vi "Move.vi"(8 "error in (no error)":errorcluster, 9 "point(x,y)":cluster{"x":i16, "y":i16}, 10 "Tools":T8=enum."Ellipse", 11 "Data in":T1={"Class"={"Ants"=refnum, "Layer"=refnum, "Templates"=refnum, "Icon"=refnum, "Glyph"=refnum, "Settings"=refnum, "Tools"=refnum, "History"=refnum}, "Ref"={"Add Layer"=refnum, "Remove Layer"=refnum, "Line Text"=[], "Body Text Spec"=refnum, "DNL_Font"=refnum, "glyph path str"=refnum, "templates path str"=refnum, "Arrow Up"=refnum, "Arrow Down"=refnum, "IE VI Ref"=refnum, "Glyphs tree"=refnum, "Templates tree"=refnum, "Layer Icon Text"=refnum, "Layer Template"=refnum, "Body Text"=refnum, "Search Templates"=refnum, "TextMarker"=refnum, "Tab Control"=refnum, "Search Glyphs"=refnum, "Line Color"=refnum, "DNL_Glyphs []"=refnum, "Fill Color"=refnum, "Tools"=refnum, "Icon"=refnum, "Preview"=refnum, "Ants"=refnum, "Terminals"=refnum, "menu reference"=refnum, "LayerNames"=[], "GlyphLoadAnimation"=refnum, "TemplateLoadAnimation"=refnum, "refreshGlyphs"=refnum, "refreshTemplates"=refnum}, "Support"={"AntsRect"={"left"=0, "top"=0, "right"=0, "bottom"=0}, "Mouse Move Coords"={"Horizontal"=0, "Vertical"=0}, "Mouse Down Coords"={"Horizontal"=0, "Vertical"=0}, "Temp Coord"={"Horizontal"=0, "Vertical"=0}, "Action"=enum."Default", "Edge Color"=4914962, "Fill Color"=16860, "Mouse Down?"=FALSE, "Draft Mode?"=FALSE, "Temp Icon"=bytes[3102], "CTRL Pressed"=FALSE, "Move Selection?"=FALSE, "AntsRect Orig"={"left"=0, "top"=0, "right"=0, "bottom"=0}, "Text"="", "TM Set?"=FALSE, "Mouse inside icon?"=FALSE, "Tool (old value)"=0, "Pencil Move Color"=0, "Swap Colors?"=FALSE, "Shift pressed?"=FALSE}}) -> (0 "error out":errorcluster, 1 "Origin":T5, 2 "Active Layer":i32, 3 "Data out":T1={"Class"={"Ants"=refnum, "Layer"=refnum, "Templates"=refnum, "Icon"=refnum, "Glyph"=refnum, "Settings"=refnum, "Tools"=refnum, "History"=refnum}, "Ref"={"Add Layer"=refnum, "Remove Layer"=refnum, "Line Text"=[], "Body Text Spec"=refnum, "DNL_Font"=refnum, "glyph path str"=refnum, "templates path str"=refnum, "Arrow Up"=refnum, "Arrow Down"=refnum, "IE VI Ref"=refnum, "Glyphs tree"=refnum, "Templates tree"=refnum, "Layer Icon Text"=refnum, "Layer Template"=refnum, "Body Text"=refnum, "Search Templates"=refnum, "TextMarker"=refnum, "Tab Control"=refnum, "Search Glyphs"=refnum, "Line Color"=refnum, "DNL_Glyphs []"=refnum, "Fill Color"=refnum, "Tools"=refnum, "Icon"=refnum, "Preview"=refnum, "Ants"=refnum, "Terminals"=refnum, "menu reference"=refnum, "LayerNames"=[], "GlyphLoadAnimation"=refnum, "TemplateLoadAnimation"=refnum, "refreshGlyphs"=refnum, "refreshTemplates"=refnum}, "Support"={"AntsRect"={"left"=0, "top"=0, "right"=0, "bottom"=0}, "Mouse Move Coords"={"Horizontal"=0, "Vertical"=0}, "Mouse Down Coords"={"Horizontal"=0, "Vertical"=0}, "Temp Coord"={"Horizontal"=0, "Vertical"=0}, "Action"=enum."Default", "Edge Color"=4914962, "Fill Color"=16860, "Mouse Down?"=FALSE, "Draft Mode?"=FALSE, "Temp Icon"=bytes[3102], "CTRL Pressed"=FALSE, "Move Selection?"=FALSE, "AntsRect Orig"={"left"=0, "top"=0, "right"=0, "bottom"=0}, "Text"="", "TM Set?"=FALSE, "Mouse inside icon?"=FALSE, "Tool (old value)"=0, "Pencil Move Color"=0, "Swap Colors?"=FALSE, "Shift pressed?"=FALSE}})   [LabVIEW 2020, in "Tools Paint.lvclass"]
uses:
  Tools Paint.lvclass
  Ants/Ants.lvclass
  FakedArray/FakedArray.lvclass
  vi.lib/LabVIEW Icon API/lv_icon/Classes/Icon/Icon.lvclass
  Icon Library/Glyph.lvclass
  Settings/Settings.lvclass
  vi.lib/LabVIEW Icon API/lv_icon/Classes/Layer/Layer.lvclass
  Tools Paint.lvclass/Tools Paint.ctl
  Controls/Circle.ctl
  Controls/Dropper.ctl
  Controls/FCircle.ctl
  Controls/Fill.ctl
  Controls/FRect.ctl
  Controls/Line.ctl
  Controls/Move.ctl
  Controls/Pen.ctl
  Controls/IERect.ctl
  Controls/Rubber.ctl
  Controls/Selection.ctl
  Controls/Text.ctl
  Controls/Tools.ctl
  <vilib>/Utility/miscctls.llb/LVPoint32TypeDef.ctl
  Controls/SupportClass_Action.ctl
  vi.lib/LabVIEW Icon API/lv_icon/Controls/IEColor.ctl
  Controls/Support Cluster.ctl
  lv_icon.lvlib
  Controls/References Cluster.ctl
  Controls/IE Classes.ctl
  Controls/Global Data.ctl
  History/History/History.lvclass
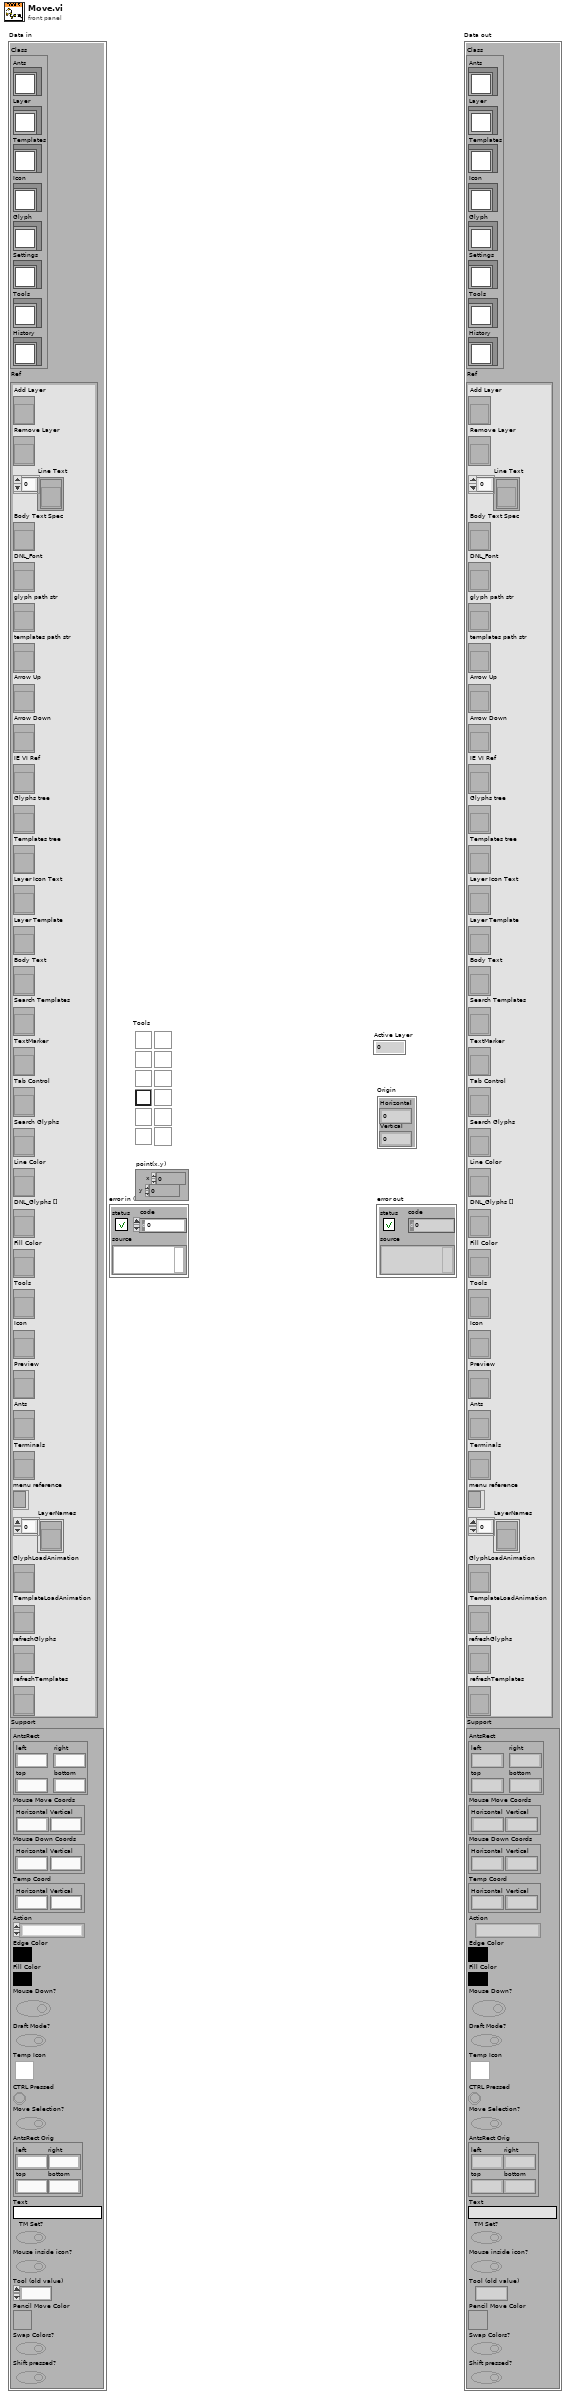
[diagram p1: front panel]
types:
  T1 = typedef "lv_icon.lvlib/Global Data.ctl" = cluster{"Class":T2, "Ref":T3, "Support":T4}
  T2 = typedef "lv_icon.lvlib/IE Classes.ctl" = cluster{"Ants":refnum<class "Ants.lvclass">, "Layer":refnum<class "FakedArray.lvclass">, "Templates":refnum<class "FakedArray.lvclass">, "Icon":refnum<class "Icon.lvclass">, "Glyph":refnum<class "Glyph.lvclass">, "Settings":refnum<class "Settings.lvclass">, "Tools":refnum<class "Tools Paint.lvclass">, "History":refnum<class "History.lvclass">}
  T3 = typedef "lv_icon.lvlib/References Cluster.ctl" = cluster{"Add Layer":refnum<vi>, "Remove Layer":refnum<vi>, "Line Text":refnum<vi>[], "Body Text Spec":refnum<vi>, "DNL_Font":refnum<vi>, "glyph path str":refnum<vi>, "templates path str":refnum<vi>, "Arrow Up":refnum<vi>, "Arrow Down":refnum<vi>, "IE VI Ref":refnum<vi>, "Glyphs tree":refnum<vi>, "Templates tree":refnum<vi>, "Layer Icon Text":refnum<vi>, "Layer Template":refnum<vi>, "Body Text":refnum<vi>, "Search Templates":refnum<vi>, "TextMarker":refnum<vi>, "Tab Control":refnum<vi>, "Search Glyphs":refnum<vi>, "Line Color":refnum<vi>, "DNL_Glyphs []":refnum<vi>, "Fill Color":refnum<vi>, "Tools":refnum<vi>, "Icon":refnum<vi>, "Preview":refnum<vi>, "Ants":refnum<vi>, "Terminals":refnum<vi>, "menu reference":refnum<k9>, "LayerNames":refnum<vi>[], "GlyphLoadAnimation":refnum<vi>, "TemplateLoadAnimation":refnum<vi>, "refreshGlyphs":refnum<vi>, "refreshTemplates":refnum<vi>}
  T4 = typedef "lv_icon.lvlib/Support Cluster.ctl" = cluster{"AntsRect":cluster{"left":i16, "top":i16, "right":i16, "bottom":i16}, "Mouse Move Coords":T5, "Mouse Down Coords":T5, "Temp Coord":T5, "Action":T6, "Edge Color":T7, "Fill Color":T7, "Mouse Down?":bool, "Draft Mode?":bool, "Temp Icon":picture, "CTRL Pressed":bool, "Move Selection?":bool, "AntsRect Orig":cluster{"left":i16, "top":i16, "right":i16, "bottom":i16}, "Text":string, "TM Set?":bool, "Mouse inside icon?":bool, "Tool (old value)":u32, "Pencil Move Color":u32, "Swap Colors?":bool, "Shift pressed?":bool}
  T5 = typedef "LVPoint32TypeDef.ctl" = cluster{"Horizontal":i32, "Vertical":i32}
  T6 = typedef "SupportClass_Action.ctl" = enum16{"Default", "Move Selection", "Glyph Library", "Tool"}
  T7 = typedef "IEColor.ctl" = u32
  T8 = typedef "Tools.ctl" = enum32{"Pencil", "Line", "Dropper", "Fill", "Rectangle", "Filled Rectangle", "Ellipse", "Filled Ellipse", "Eraser", "Text", "Select", "Move"}
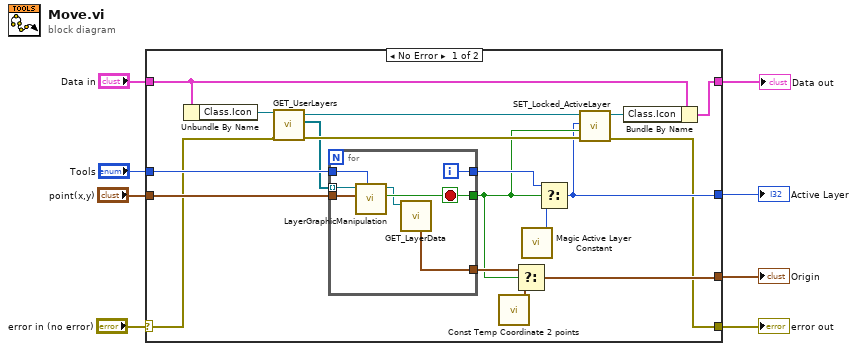
[diagram p0: block diagram]
diagram:
  n1 = case shown="No Error" "error in (no error)" {
    selector: "error in (no error)" -> [w13 w35]
    tunnel: [w9 w35] -> w7
    tunnel: "Tools" -> [w26 _]
    tunnel: "point(x,y)" -> [w25 _]
    tunnel: [w16 _] -> w4
    tunnel: [w24 _] -> w3
    tunnel: "Data in" -> [w12 w34]
    tunnel: [w10 w34] -> w1
    frame No Error {
      n2 = Unbundle By Name(w12) -> ("Class.Icon"=w14:refnum<class "Icon.lvclass">)
      n3 = call-dynamic "GET_UserLayers.vi"("error in (no error)"=w13, "Icon.lvclass in"=w14) -> ("error out"=w21:errorcluster, "All Layers"=w18:refnum<class "Layer.lvclass">[], "Icon.lvclass out"=w22:refnum<class "Icon.lvclass">)  [unwired: 7 out]
      n4 = for {
        tunnel: w26 -> [w33]
        tunnel: w25 -> [w32]
        tunnel: w18 -> [w31] mode=indexing
        tunnel: [w30] -> w17
        tunnel: [w29] -> w23
        tunnel: [w27] -> w20
        i -> [w29]
        stop <- w30 stop-if-true
        n5 = call "LayerGraphicManipulation.vi"("Radio Buttons"=w33, "point(x,y)"=w32, "Layer.lvclass"=w31) -> ("Operation processed?"=w30:bool, "Layer.lvclass out"=w28:refnum<class "Layer.lvclass">)  [unwired: 3 in, 4 out]
        n6 = call-dynamic "GET_LayerData.vi"("Layer.lvclass in"=w28) -> ("Origin"=w27:T5)  [unwired: 1 in, 9 out]
      }
      n7 = call "Const Temp Coordinate 2 points.vi"() -> ("Const Temp Coordinate"=w19:T5)  [unwired: 11 out]
      n8 = Select(t=w20, s=w17, f=w19) -> (s? t:f=w24:T5)
      n9 = call "Magic Active Layer Constant.vi"() -> ("Magic Constant"=w15:i32)  [unwired: 19 out]
      n10 = Select(t=w23, s=w17, f=w15) -> (s? t:f=w16:i32)
      n11 = call-dynamic "SET_Locked_ActiveLayer.vi"("error in (no error)"=w21, "Layers Locked?"=w17, "Active Layer"=w16, "Icon.lvclass in"=w22) -> ("error out"=w9:errorcluster, "Icon.lvclass out"=w11:refnum<class "Icon.lvclass">)  [unwired: 6 out]
      n12 = Bundle By Name(cluster=w12, "Class.Icon"=w11) -> (w10:T1)
    }
    frame Error {
    }
  }
  "error out" <- w7
  "Active Layer" <- w4
  "Origin" <- w3
  "Data out" <- w1
